vi "U8_Arr_To_I64.vi"(1 "data":u8[](array[numeric]) format="%02x") -> (0 "I64":i64 format="%01x")   [LabVIEW 2011]
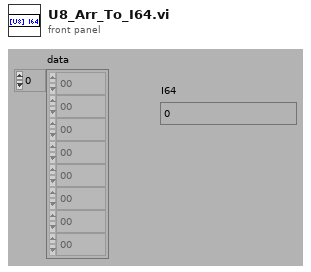
[diagram p1: front panel]
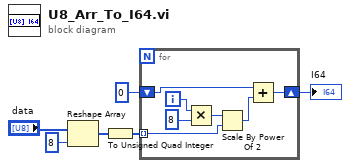
[diagram p0: block diagram]
diagram:
  n1 = Reshape Array("data", 8 ("维数大小")) -> (w1:u8[])
  n2 = To Unsigned Quad Integer(1:w1) -> (0:w4:u64[])
  n3 = for {
    tunnel: w4 -> [w10] mode=indexing
    shift-right: [w7] -> w5
    shift-left: u64 0 ("I64") -> [w9]
    i -> [w13]
    n4 = Multiply(x=w13, y=8) -> (x*y=w11:i32)
    n5 = Scale By Power Of 2(n=w11, x=w10) -> (x*2^n=w8:u64)
    n6 = Add(x=w9, y=w8) -> (x+y=w7:u64)
  }
  "I64" <- w5
